vi "module information (scan interface).vi"(8 "error in":errorcluster, 9 "number of slots":i32, 11 "IP address (localhost)":string) -> (0 "error out":errorcluster, 2 "module information":T1[](array[typedef]) {"product ID" format="%.0x"})   [LabVIEW 2014, in "SMI.lvlib" / "C Series Module.lvclass"]
uses:
  C Series Module.lvclass
  Module/module information.ctl
  <vilib>/regexp/Match Regular Expression.xnode
  <resource>/objmgr/ni.var.rc
  Module/Module.lvclass
  <resource>/objmgr/cRIO.rc
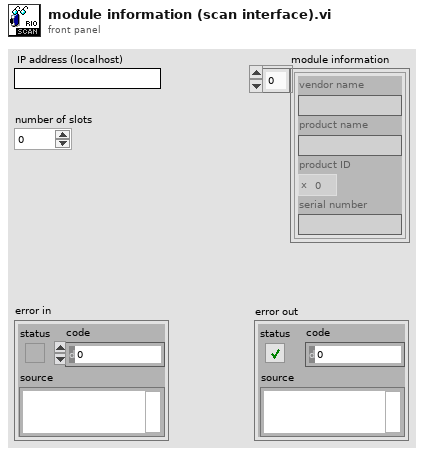
[diagram p1: front panel]
types:
  T1 = typedef "SMI.lvlib/Module.lvclass/module information.ctl" = cluster{"vendor name":string, "product name":string, "product ID":u16, "serial number":string}
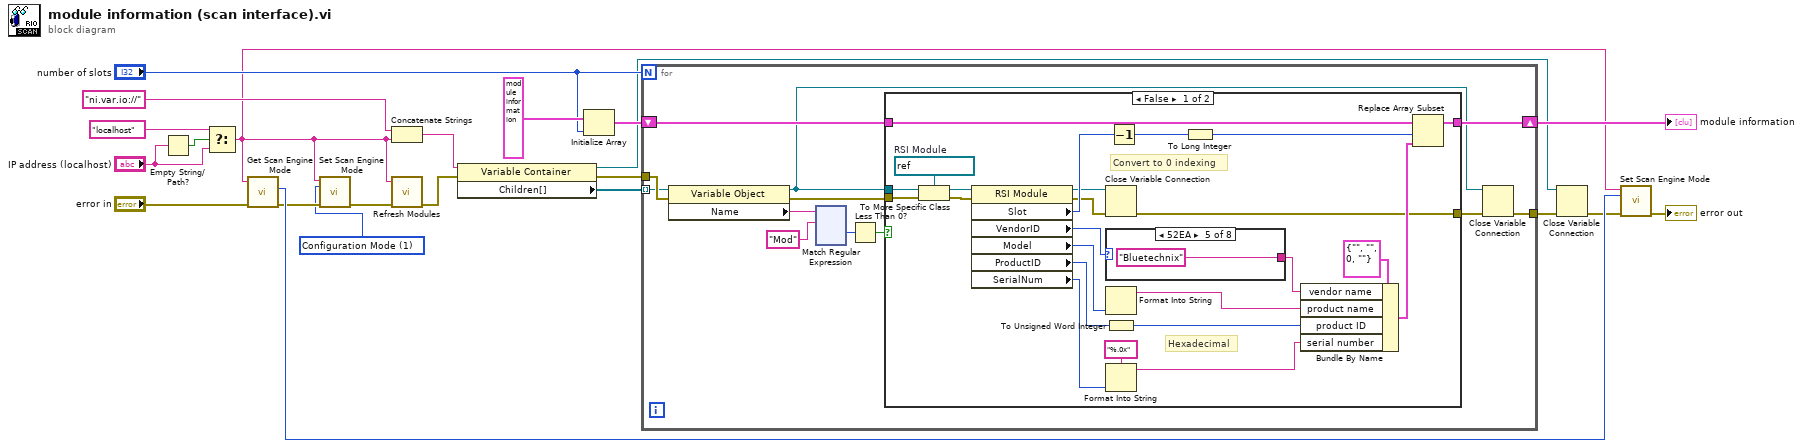
[diagram p0: block diagram]
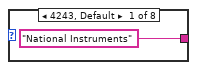
[diagram p2: hidden frame]
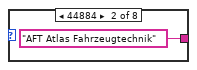
[diagram p3: hidden frame]
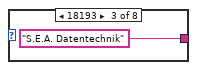
[diagram p4: hidden frame]
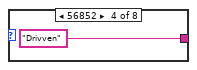
[diagram p5: hidden frame]
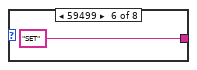
[diagram p6: hidden frame]
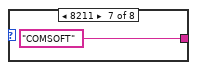
[diagram p7: hidden frame]
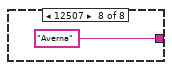
[diagram p8: hidden frame]
diagram:
  w3 = 1 items=["Initialization Mode", "Configuration Mode", "Active Mode", "Fault Mode"] ("mode")
  n1 = Empty String/Path?(string/path="IP address (localhost)") -> (empty?=w19:bool)
  n2 = Select(t="localhost" ("Resource 2"), s=w19, f="IP address (localhost)") -> (s? t:f=w2:string)
  n3 = call <vilib>:"Get Scan Engine Mode.vi"("error in (no error)"="error in", "target address (localhost)"=w2) -> ("error out"=w4:errorcluster, "mode"=w7:i32)  [unwired: 8 in]
  n4 = call <vilib>:"Set Scan Engine Mode.vi"("target address (localhost)"=w2, "mode (Active Mode)"=w3, "error in (no error)"=w4) -> ("error out"=w1:errorcluster)  [unwired: 12 in]
  n5 = Concatenate Strings("ni.var.io://" ("Resource 2"), w2) -> (w15:string)
  n6 = call <vilib>:"Refresh Modules.vi"("error in (no error)"=w1, "target address (localhost)"=w2) -> ("error out"=w20:errorcluster)  [unwired: 9 in]
  n7 = property class="Variable Container"(reference=w15, error in=w20) -> (reference out=w11:refnum<k21>, error out=w21:errorcluster, "Children[]"=w10:refnum<k21>[])
  n8 = Initialize Array(T1 {"vendor name"="Not Present", "product name"="N/A", "product ID"=0, "serial number"="N/A"} ("cRIO Module Information"), "number of slots") -> (w12:T1[])
  n9 = for {
    N: "number of slots" -> [_]
    tunnel: w10 -> [w26] mode=indexing
    tunnel: w21 -> [w28]
    tunnel: [w24] -> w9
    shift-right: [w31] -> w22
    shift-left: w12 -> [w30]
    n10 = property class="Variable Object"(reference=w26, error in=w28) -> (reference out=w25:refnum<k21>, error out=w27:errorcluster, "Name"=w32:string)
    n11 = xnode "Match Regular Expression"("input string"=w32, "regular expression"="Mod") -> ("offset past match"=w34:i32)  [unwired: 4 in, 4 out]
    n12 = Less Than 0?(x=w34) -> (x < 0?=w29:bool)
    n13 = case shown="False" w29 {
      tunnel: w27 -> [w57 w67]
      tunnel: w25 -> [w56 _]
      tunnel: [w45 w67] -> w23
      tunnel: [w55 w68] -> w31
      tunnel: w30 -> [w54 w68]
      frame False {
        w58 = refnum<k21> refnum  # RSI Module
        # "Hexadecimal"
        # "Convert to 0 indexing"
        n14 = To More Specific Class(target class=w58, reference=w56, error in=w57) -> (specific class reference=w53:refnum<k21>, error out=w52:errorcluster)
        n15 = property class="RSI Module"(reference=w53, error in=w52) -> (reference out=w47:refnum<k21>, error out=w46:errorcluster, "Slot"=w50:u32, "VendorID"=w43:u32, "Model"=w41:u32, "ProductID"=w39:u32, "SerialNum"=w37:u32)
        n16 = Close Variable Connection(8:w46, 11:w47) -> (0:w45:errorcluster)
        n17 = case shown="52EA" w43 {
          tunnel: ["National Instruments" "AFT Atlas Fahrzeugtechnik" "S.E.A. Datentechnik" "Drivven" "Bluetechnix" "SET" "COMSOFT" "Averna"] -> w42
          frame 4243, Default {
          }
          frame 44884 {
          }
          frame 18193 {
          }
          frame 56852 {
          }
          frame 21226 {
          }
          frame 59499 {
          }
          frame 8211 {
          }
          frame 12507 {
          }
        }
        n18 = Format Into String(w41) -> (resulting string=w40:string)  [unwired: 3 in, 1 out]
        n19 = To Unsigned Word Integer(number=w39) -> (unsigned 16bit integer=w38:u16)
        n20 = Format Into String(format string="%.0x", w37) -> (resulting string=w36:string)  [unwired: 2 in, 1 out]
        n21 = Decrement(x=w50) -> (x-1=w44:u32)
        n22 = To Long Integer(number=w44) -> (32bit integer=w49:i32)
        n23 = Bundle By Name(cluster=T1 {"vendor name"="", "product name"="", "product ID"=0, "serial number"=""} ("cRIO Module Information"), "vendor name"=w42, "product name"=w40, "product ID"=w38, "serial number"=w36) -> (w48:T1)
        n24 = Replace Array Subset(array=w54, new element=w48, index=w49) -> (w55:T1[])
      }
      frame True {
        # "The Variable Object is not a module"
      }
    }
    n25 = Close Variable Connection(8:w23, 11:w25) -> (0:w24:errorcluster)
  }
  "module information" <- w22
  n26 = Close Variable Connection(8:w9, 11:w11) -> (0:w6:errorcluster)
  n27 = call <vilib>:"Set Scan Engine Mode.vi"("target address (localhost)"=w2, "mode (Active Mode)"=w7, "error in (no error)"=w6) -> ("error out"=→"error out":errorcluster)  [unwired: 12 in]
